vi "c_ctre_phoenix6_orchestra_AddDevice.vi"(0 "Numeric 2":u16, 1 "String":string, 2 "Numeric 3":u32) -> (20 "Numeric":i32)   [LabVIEW 2023]
uses:
  <vilib>/Rock Robotics/WPI/ThirdParty/Phoenix-LabVIEW/Controls/DriverLib.ctl
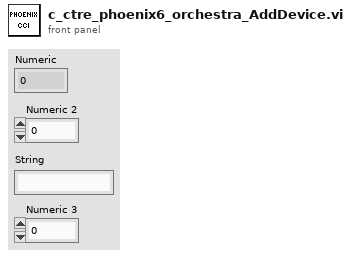
[diagram p1: front panel]
types:
  T1 = typedef "DriverLib.ctl" = path
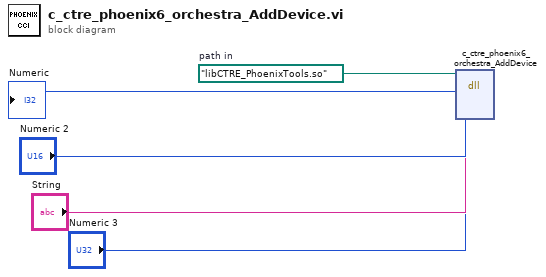
[diagram p0: block diagram]
diagram:
  w5 = T1 path "libCTRE_PhoenixTools.so"  # path in
  n1 = dll-call lib="?" fn="c_ctre_phoenix6_orchestra_AddDevice"(path in=w5, "Numeric 2", "String", "Numeric 3") -> (→"Numeric":i32)  [unwired: 5 in, 2 out]
